vi "Collect Data V1.00.vi"(1 "McP Scan Parameter":T1={"McP on?"=TRUE, "Wait"=0.0, "X-Axis Unit String"="", "Data Format"=1, "Scanning Pattern:"=0, "Spex on?"=TRUE} {"Scanning Pattern:" items=["Uniform Points ", "User Defined Point Pattern ", "Time-Drive"]; "Data Format" items=["Original", "1024rows X 2cloumns", "Future Use"]; "Wait" format="%.2f"}, 2 "Scaling Factors":dbl[](array[numeric]) format="%.2f", 3 "input limits (no change)":T2(array[cluster]) {"low limit (-10V)" format="%.2f"; "high limit (10V)" format="%.2f"}, 5 "Point Number":i32, 6 "stop":bool, 7 "channels (0)":string[](array[string])=["0"], 8 "Number of Channels":i16, 9 "Number to Average":i32=32, 10 "Board Number":i16=4) -> (0 "Output Data":dbl[](array[numeric]) format="%.2e", 4 "Stop":bool)   [LabVIEW 2020]
doc: "Reads the analog inputs, averages the values, reads the GPIB instruments and outputs all the values in a single 1D array.\nScott Hannahs, NHMFLL, Sept 1993"
uses:
  McP Parameter.ctl
  <vilib>/Analysis/baseanly.llb/Mean (DBL).vi
  <vilib>/Analysis/NI_AALBase.lvlib
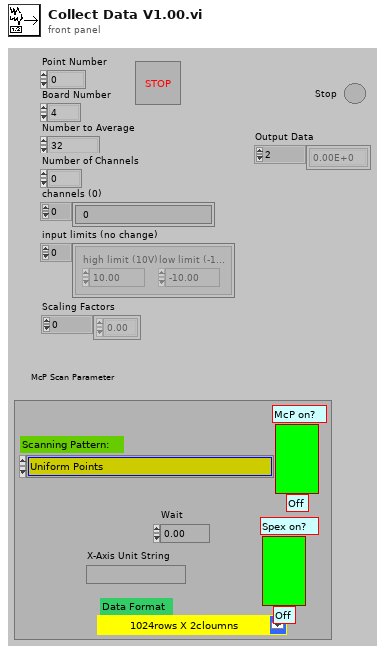
[diagram p1: front panel]
types:
  T1 = typedef "McP Parameter.ctl" = cluster{"McP on?":bool, "Wait":dbl, "X-Axis Unit String":string, "Data Format":u8, "Scanning Pattern:":u32, "Spex on?":bool}
  T2 = cluster{"high limit (10V)":sgl, "low limit (-10V)":sgl}[]
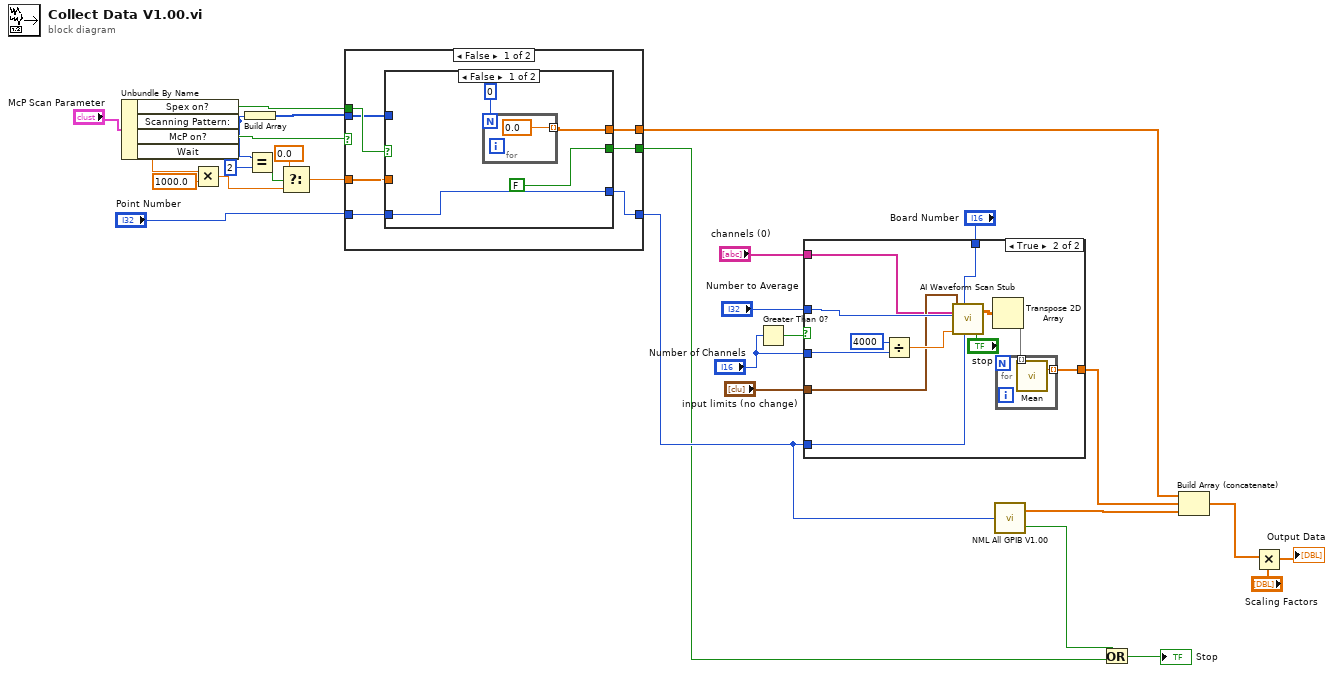
[diagram p0: block diagram]
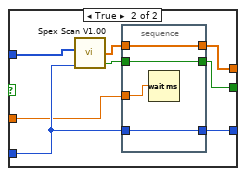
[diagram p2: hidden frame]
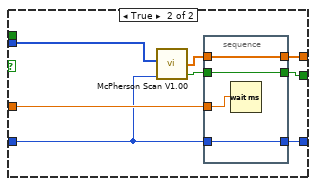
[diagram p3: hidden frame]
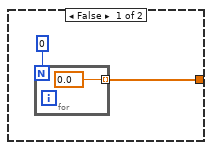
[diagram p4: hidden frame]
diagram:
  n1 = Unbundle By Name("McP Scan Parameter") -> ("Spex on?"=w1:bool, "Scanning Pattern:"=w7:u32, "McP on?"=w17:bool, "Wait"=w9:dbl)
  n2 = Multiply(x=w9, y=1000.0) -> (x*y=w4:dbl)
  n3 = Build Array(w7) -> (w8:u32[])
  n4 = Equal?(x=w7, y=u32 2) -> (x = y?=w5:bool)
  n5 = Select(t=0.0, s=w5, f=w4) -> (s? t:f=w2:dbl)
  n6 = case shown="False" w17 {
    tunnel: [w36 w59] -> w18
    tunnel: w8 -> [w30 w61]
    tunnel: "Point Number" -> [w33 w55]
    tunnel: [w32 w54] -> w15
    tunnel: [w35 w57] -> w12
    tunnel: w2 -> [w31 w56]
    tunnel: w1 -> [w34 _]
    frame False {
      n7 = case shown="False" w34 {
        tunnel: [w39 w43] -> w36
        tunnel: [FALSE ("Stop") w42] -> w35
        tunnel: w33 -> [w37 w47]
        tunnel: [w37 w46] -> w32
        tunnel: w31 -> [_ w45]
        tunnel: w30 -> [_ w44]
        frame False {
          n8 = for {
            N: 0 -> [_]
            tunnel: [0.0] -> w39 mode=indexing
          }
        }
        frame True {
          n9 = call "Spex Scan V1.00.vi"("Point #"=w47, "Parameters"=w44) -> ("Stop"=w48:bool, "Data Out"=w49:dbl[])  [unwired: 3 in]
          n10 = stacked-sequence {
            tunnel: w49 -> [w53]
            tunnel: [w53] -> w43
            tunnel: w48 -> [w52]
            tunnel: [w52] -> w42
            tunnel: w45 -> [w51]
            tunnel: w47 -> [w50]
            tunnel: [w50] -> w46
            frame #0 {
              n11 = Wait (ms)(milliseconds to wait=w51) -> ()  [unwired: 1 out]
            }
          }
        }
      }
    }
    frame True {
      n12 = call "McPherson Scan V1.00.vi"("Point #"=w55, "Parameters"=w61) -> ("Stop"=w58:bool, "Data Out"=w60:dbl[])  [unwired: 3 in]
      n13 = stacked-sequence {
        tunnel: w60 -> [w65]
        tunnel: [w65] -> w59
        tunnel: w58 -> [w64]
        tunnel: [w64] -> w57
        tunnel: w56 -> [w63]
        tunnel: w55 -> [w62]
        tunnel: [w62] -> w54
        frame #0 {
          n14 = Wait (ms)(milliseconds to wait=w63) -> ()  [unwired: 1 out]
        }
      }
    }
  }
  n15 = Greater Than 0?(x="Number of Channels") -> (x > 0?=w25:bool)
  n16 = case shown="True" w25 {
    tunnel: w15 -> [_ w77]
    tunnel: "Board Number" -> [_ w78]
    tunnel: "Number to Average" -> [_ w79]
    tunnel: "input limits (no change)" -> [_ w72]
    tunnel: "Number of Channels" -> [_ w80]
    tunnel: [w66 w73] -> w21
    tunnel: "channels (0)" -> [_ w71]
    frame False {
      n17 = for {
        N: 0 -> [_]
        tunnel: [0.0] -> w66 mode=indexing
      }
    }
    frame True {
      n18 = Divide(x=4000, y=w80) -> (x/y=w76:dbl)
      n19 = call "AI Waveform Scan Stub.vi"("stop"="stop", "Point Number"=w77, "Board Number"=w78, "Numeric"=w76, "input limits (no change)"=w72, "Number to Average"=w79, "channels (0)"=w71) -> ("scaled data"=w74:sgl[][])
      n20 = Transpose 2D Array(2D array=w74) -> (transposed array=w69:sgl[][])
      n21 = for {
        tunnel: w69 -> [w82] mode=indexing
        tunnel: [w81] -> w73 mode=indexing
        n22 = call-poly <vilib>:"Mean.vi"("X"=w82) -> ("mean"=w81:dbl)  [unwired: 1 out]
      }
    }
  }
  n23 = call "NML All GPIB V1.00.vi"("Point #"=w15) -> ("GPIB Data Out"=w22:dbl[], "Stop Out"=w14:bool)
  n24 = Or(x=w14, y=w12) -> (x .or. y?=→"Stop":bool)
  n25 = Build Array (concatenate)(w18, w21, w22) -> (w19:dbl[])
  n26 = Multiply(x=w19, y="Scaling Factors") -> (x*y=→"Output Data":dbl[])
